vi "Finalize.vi"(8 "error in (no error)":errorcluster, 11 "Results in":refnum<class "Results.lvclass">) -> (0 "error out":errorcluster, 2 "Overall Result":T1, 3 "Results out":refnum<class "Results.lvclass">)   [LabVIEW 2020, in "Tester.lvlib" / "Results.lvclass"]
uses:
  Results.lvclass
  Result.ctl
  Results.lvclass/Results.ctl
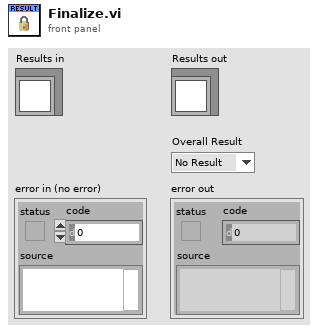
[diagram p1: front panel]
types:
  T1 = typedef "Tester.lvlib/Results.lvclass/Result.ctl" = enum16{"No Result", "Pass", "Fail", "Error", "Abort"}
  T2 = typedef "Tester.lvlib/Results.lvclass/Results Ref.ctl" = cluster{"Entries":T3[], "Overall Result":T1}
  T3 = typedef "Tester.lvlib/Results.lvclass/Entry.ctl" = cluster{"Name":string, "Value":variant, "Result":T1}
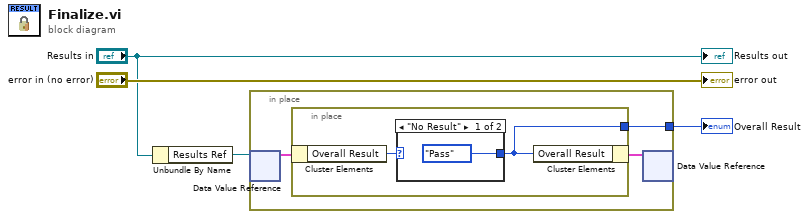
[diagram p0: block diagram]
diagram:
  n1 = Unbundle By Name("Results in") -> ("Results Ref"=w3:refnum<data-value>)
  n2 = in-place {
    in-place-border: [w5] -> w1
    n3 = in-place-dvr #1(w3) -> (w7:T2)  [unwired: 1 out]
    n4 = in-place {
      in-place-border: [w8] -> w5
      n5 = in-place-cluster #2(w7) -> ("Overall Result"=w9:T1)
      n6 = case shown="\"No Result\"" w9 {
        selector: w9 -> [_ w11]
        tunnel: [Result."Pass" ("Overall Result") w11] -> w8
        frame "No Result" {
        }
        frame Default {
        }
      }
      n7 = in-place-cluster #2("Overall Result"=w8) -> (w6:T2)
    }
    n8 = in-place-dvr #1(w6) -> ()  [unwired: 2 out]
  }
  "Overall Result" <- w1
  "error out" <- "error in (no error)"
  "Results out" <- "Results in"
